vi "FormatTracePointsServerString.vi"(8 "error in":errorcluster, 11 "TracePointName":string) -> (0 "error out":errorcluster, 1 "Message out":T1)   [LabVIEW 2017, in "TracePointSynchronizer.lvlib"]
uses:
  <vilib>/addons/InsightCM/Devices/Shared/Common/TracePointSynchronizer/TracePointSynchronizer.lvlib
  <vilib>/addons/InsightCM/MessageBus/Base/controls/Message.ctl
  <vilib>/addons/InsightCM/MessageBus/Base/controls/MessageHeader.ctl
  <vilib>/addons/InsightCM/MessageBus/Base/controls/KeyValuePair.ctl
  <vilib>/addons/InsightCM/MessageBus/MessageLibrary/TraceLogger/controls/TraceLoggerRegisterTracePointRoutedMessageBody.ctl
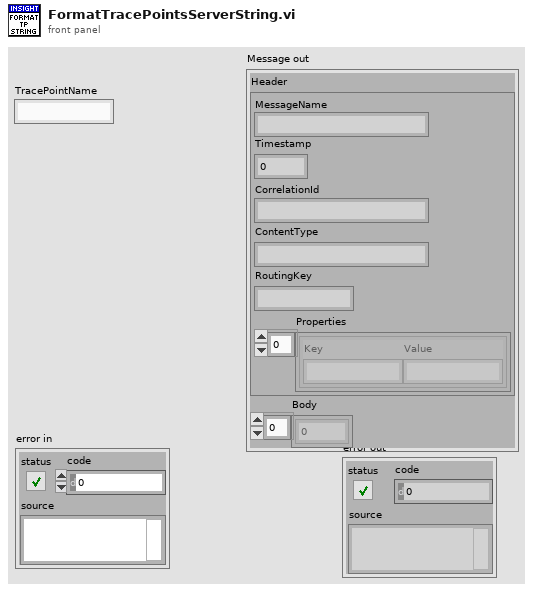
[diagram p1: front panel]
types:
  T1 = typedef "Message.ctl" = cluster{"Header":T2, "Body":u8[]}
  T2 = typedef "MessageHeader.ctl" = cluster{"MessageName":string, "Timestamp":i64, "CorrelationId":string, "ContentType":string, "RoutingKey":string, "Properties":T3[]}
  T3 = typedef "KeyValuePair.ctl" = cluster{"Key":string, "Value":string}
  T4 = typedef "TraceLoggerRegisterTracePointRoutedMessageBody.ctl" = cluster{"TracePointName":string}
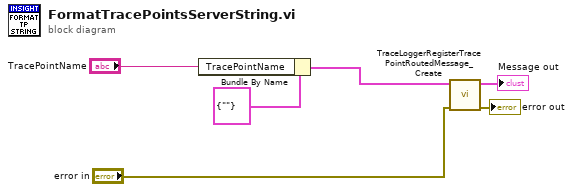
[diagram p0: block diagram]
diagram:
  n1 = Bundle By Name(cluster=T4 {"TracePointName"=""} ("Body"), "TracePointName"="TracePointName") -> (w1:T4)
  n2 = call <vilib>:"TraceLoggerRegisterTracePointRoutedMessage_Create.vi"("error in (no error)"="error in", "TraceLoggerRegisterTracePointRoutedMessage"=w1) -> ("error out"=→"error out":errorcluster, "Message"=→"Message out":T1)  [unwired: 8 in]
